vi "CMD_Shoot.vi"(1 "Line":string) -> (0 "Done":bool)   [LabVIEW 2013]
panel:
  in  "Parameters":i32[](array[numeric])=[0, 0, 0, 1]
  in  "Subcommands":string[](array[string])=["", "continue", "finish", "until"]
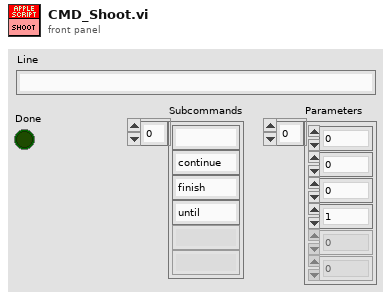
[diagram p1: front panel]
types:
  T1 = enum16{"Wait", "Clear", "Release", "Cock", "Reset"}
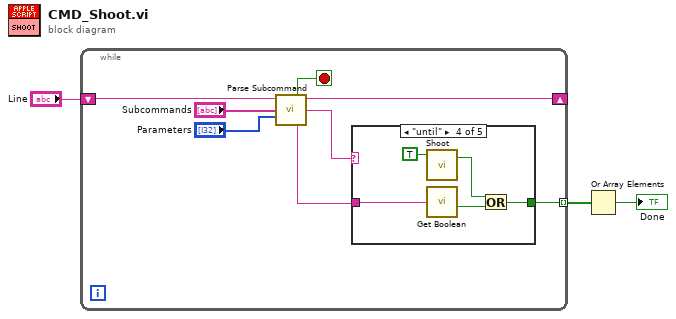
[diagram p0: block diagram]
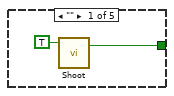
[diagram p2: hidden frame]
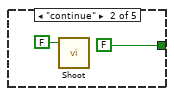
[diagram p3: hidden frame]
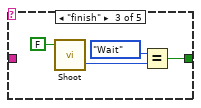
[diagram p4: hidden frame]
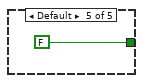
[diagram p5: hidden frame]
diagram:
  n1 = while {
    shift-right: [w8] -> _
    shift-left: "Line" -> [w11]
    tunnel: [w5] -> w1 mode=indexing
    stop <- w7 stop-if-true
    n2 = call "Parse Subcommand.vi"("Text In"=w11, "Subcommands"="Subcommands", "Parameters"="Parameters") -> ("Done"=w7:bool, "Text Out"=w8:string, "Subcommand"=w6:string, "Parameter 1"=w4:string)  [unwired: 6 in, 3 out]
    n3 = case shown="\"until\"" w6 {
      tunnel: [w12 FALSE ("Finished Cycle") w16 w22 FALSE ("Finished Cycle")] -> w5
      tunnel: w4 -> [_ _ _ w24 _]
      frame "" {
        n4 = call "Shoot.vi"("Shoot"=TRUE) -> ("Finished Cycle"=w12:bool)  [unwired: 3 in, 1 out]
      }
      frame "continue" {
        n5 = call "Shoot.vi"("Shoot"=FALSE) -> ()  [unwired: 3 in, 2 out]
      }
      frame "finish" {
        n6 = call "Shoot.vi"("Shoot"=FALSE) -> ("State"=w17:T1)  [unwired: 3 in, 1 out]
        n7 = Equal?(x=T1."Wait", y=w17) -> (x = y?=w16:bool)
      }
      frame "until" {
        n8 = call "Shoot.vi"("Shoot"=TRUE) -> ("Finished Cycle"=w21:bool)  [unwired: 3 in, 1 out]
        n9 = call "Get Boolean.vi"("Name"=w24) -> ("Value"=w20:bool)
        n10 = Or(x=w21, y=w20) -> (x .or. y?=w22:bool)
      }
      frame Default {
      }
    }
  }
  n11 = Or Array Elements(Boolean array=w1) -> (logical OR=→"Done":bool)
